vi "ev Frame num.vi"(8 "error in (no error)":errorcluster, 11 "IDE simple in":refnum<class "Main Panel.lvclass">) -> (0 "error out":errorcluster, 3 "IDE simple out":refnum<class "Main Panel.lvclass">)   [LabVIEW 2018, in "Main Panel.lvlib" / "Main Panel.lvclass"]
uses:
  Main Panel.lvclass
  Main Panel.lvclass/Main Panel.ctl
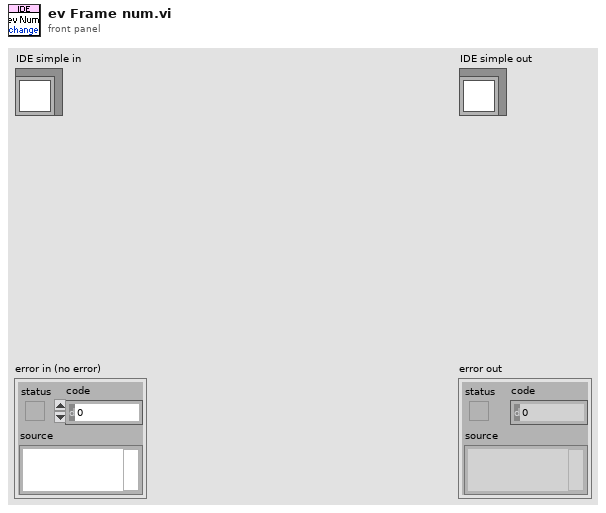
[diagram p1: front panel]
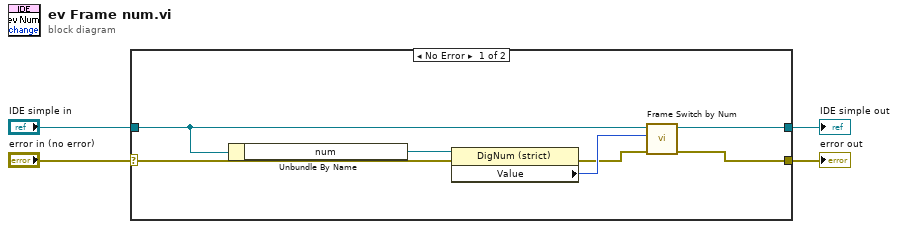
[diagram p0: block diagram]
diagram:
  n1 = case shown="No Error" "error in (no error)" {
    selector: "error in (no error)" -> [w10 w13]
    tunnel: [w5 w13] -> w3
    tunnel: [w6 w12] -> w1
    tunnel: "IDE simple in" -> [w9 w12]
    frame No Error {
      n2 = Unbundle By Name(w9) -> ("num"=w11:refnum<vi>)
      n3 = property class="DigNum (strict)"(reference=w11, error in=w10) -> (error out=w7:errorcluster, "Value"=w8:u32)  [unwired: 1 out]
      n4 = call "Frame Switch by Num.vi"("error in (no error)"=w7, "Frame Num"=w8, "LF2R IDE in"=w9) -> ("error out"=w5:errorcluster, "LF2R IDE out"=w6:refnum<class "Main Panel.lvclass">)  [unwired: 7 in]
    }
    frame Error {
    }
  }
  "error out" <- w3
  "IDE simple out" <- w1
